vi "Reinitialize.vi"(8 "error in (no error)":errorcluster, 11 "VGC in":refnum<class "PL Inficon VGC.lvclass">) -> (0 "error out":errorcluster, 3 "VGC out":refnum<class "PL Inficon VGC.lvclass">)   [LabVIEW 2015, in "PL Inficon VGC.lvclass"]
doc: "Reinitializes connection to device based on previously specified settings."
uses:
  PL Inficon VGC.lvclass
  PL Inficon VGC.lvclass/PL Inficon VGC.ctl
  <vilib>/Instr/_visa.llb/VISA Configure Serial Port (Instr).vi
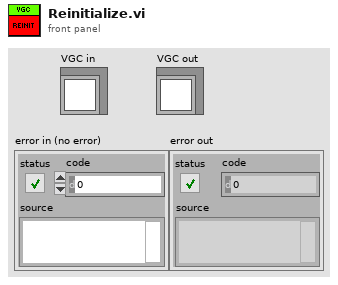
[diagram p1: front panel]
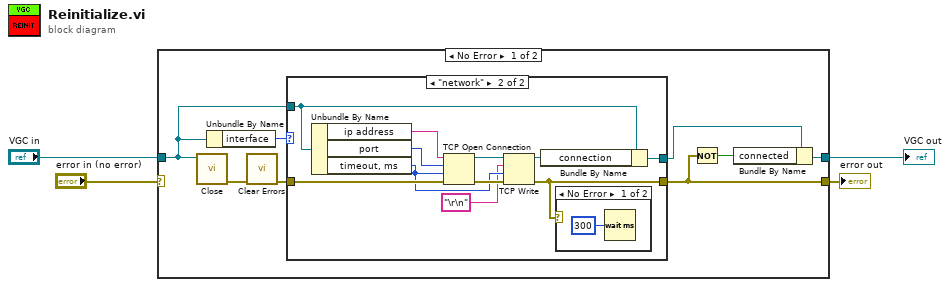
[diagram p0: block diagram]
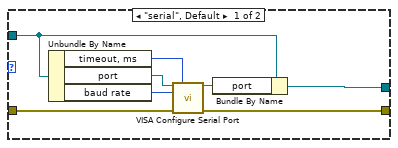
[diagram p2: hidden frame]
diagram:
  n1 = case shown="No Error" "error in (no error)" {
    selector: "error in (no error)" -> [_ w33]
    tunnel: "VGC in" -> [w5 w34]
    tunnel: [w9 w34] -> w3
    tunnel: [w8 w33] -> w2
    frame No Error {
      n2 = call "Close.vi"("VGC in"=w5) -> ("error out"=w6:errorcluster)  [unwired: 10 in]
      n3 = Unbundle By Name(w5) -> ("interface"=w12:enum16{"serial", "network"})
      n4 = call <vilib>:"Clear Errors.vi"("error in (no error)"=w6) -> ("error out"=w7:errorcluster)  [unwired: 5 in, 1 out]
      n5 = case shown="\"network\"" w12 {
        tunnel: [w16 w21] -> w8
        tunnel: [w20 w31] -> w11
        tunnel: w5 -> [w19 w30]
        tunnel: w7 -> [w14 w29]
        frame "serial", Default {
          n6 = Unbundle By Name(w19) -> ("timeout, ms"=w13:u32, "port"=w15:refnum<visa-resource-name>, "baud rate"=w18:u32)
          n7 = call-poly "VISA Configure Serial Port"("VISA resource name"=w15, "timeout (10sec)"=w13, "baud rate (9600)"=w18, "error in (no error)"=w14) -> ("VISA resource name out"=w17:refnum<visa-resource-name>, "error out"=w16:errorcluster)  [unwired: 10 in]
          n8 = Bundle By Name(cluster=w19, "port"=w17) -> (w20:refnum<class "PL Inficon VGC.lvclass">)
        }
        frame "network" {
          n9 = Unbundle By Name(w30) -> ("ip address"=w27:string, "port"=w28:u16, "timeout, ms"=w24:u32)
          n10 = TCP Open Connection(address=w27, remote port or service name=w28, timeout ms (60000)=w24, error in (no error)=w29) -> (connection ID=w26:refnum<k5>, error out=w25:errorcluster)  [unwired: 1 in]
          n11 = TCP Write(connection ID=w26, data in="\r\n" ("string"), error in (no error)=w25, 9:w24) -> (connection ID out=w22:refnum<k5>, error out=w21:errorcluster)  [unwired: 1 out]
          n12 = Bundle By Name(cluster=w30, "connection"=w22) -> (w31:refnum<class "PL Inficon VGC.lvclass">)
          n13 = case shown="No Error" w21 {
            frame No Error {
              n14 = Wait (ms)(milliseconds to wait=u32 300) -> ()  [unwired: 1 out]
            }
            frame Error {
            }
          }
        }
      }
      n15 = Not(x=w8) -> (.not. x?=w10:bool)
      n16 = Bundle By Name(cluster=w11, "connected"=w10) -> (w9:refnum<class "PL Inficon VGC.lvclass">)
    }
    frame Error {
    }
  }
  "VGC out" <- w3
  "error out" <- w2
